vi "from string.vi"(8 "error in":errorcluster, 9 "data":string, 10 "version":string, 11 "TEC configuration in":refnum<class "TEC configuration.lvclass">) -> (0 "error out":errorcluster, 3 "TEC configuration out":refnum<class "TEC configuration.lvclass">)   [LabVIEW 2013, in "TEC configuration.lvclass"]
doc: "Provides an interface for loading a module configuration from a file or other serialized data source. It is recommended that all children of this class store data in two sets--data required for its own initialization, and any data required for parent initialization--and that each implementation uses the <b>Call Parent Method</b> primitive to de-serialize parent information. As a result, it is expected that every module configuration class calls <b>component configuration.lvclass:From String.vi</b>."
uses:
  TEC configuration.lvclass
  <vilib>/NI/Tag Bus Module Framework/channel/TBM channel.lvclass
  <vilib>/NI/Tag Bus Module Framework/module configuration/TBM module configuration.lvclass
  TEC configuration.lvclass/TEC configuration.ctl
  <vilib>/NI/Tag Bus Module Framework/root configuration/TBM configuration.lvclass
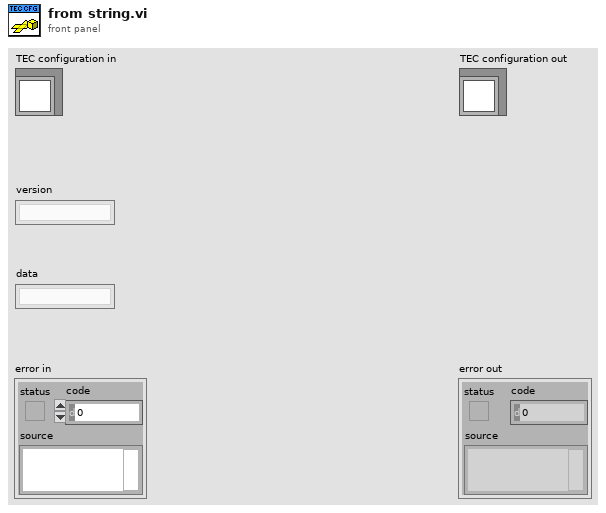
[diagram p1: front panel]
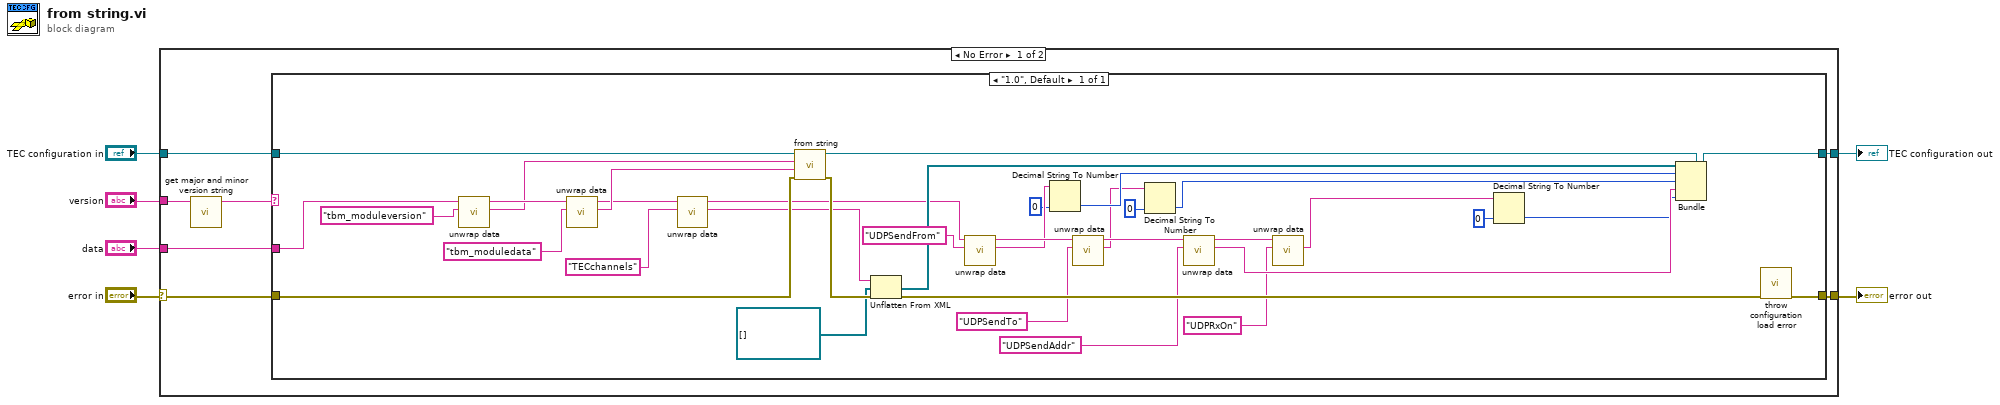
[diagram p0: block diagram]
diagram:
  n1 = case shown="No Error" "error in" {
    selector: "error in" -> [w7 w51]
    tunnel: "data" -> [w13 _]
    tunnel: "TEC configuration in" -> [w12 w50]
    tunnel: [w11 w50] -> w5
    tunnel: [w10 w51] -> w4
    tunnel: "version" -> [w9 _]
    frame No Error {
      n2 = call <vilib>:"get major and minor version string.vi"("full version"=w9) -> ("major.minor version"=w8:string)  [unwired: 10 in]
      n3 = case shown="\"1.0\", Default" w8 {
        tunnel: w13 -> [w44]
        tunnel: w7 -> [w43]
        tunnel: w12 -> [w49]
        tunnel: [w38] -> w11
        tunnel: [w46] -> w10
        frame "1.0", Default {
          n4 = call <vilib>:"unwrap data.vi"("identifier"="tbm_moduleversion" ("additional identifier"), "data to unwrap"=w44) -> ("unwrapped data"=w39:string, "remaining string"=w45:string)  [unwired: 8 in]
          n5 = call <vilib>:"unwrap data.vi"("identifier"="tbm_moduledata" ("additional identifier"), "data to unwrap"=w45) -> ("unwrapped data"=w41:string, "remaining string"=w34:string)  [unwired: 8 in]
          n6 = call <vilib>:"unwrap data.vi"("identifier"="TECchannels" ("additional identifier"), "data to unwrap"=w34) -> ("unwrapped data"=w32:string, "remaining string"=w28:string)  [unwired: 8 in]
          n7 = call-parent "from string.vi"("error in"=w43, "data"=w41, "version"=w39, "module configuration in"=w49) -> ("error out"=w47:errorcluster, "module configuration out"=w48:refnum<class "TEC configuration.lvclass">)  [unwired: 6 in]
          n8 = Unflatten From XML(xml string=w32, type=refnum<class "TBM channel.lvclass">[] [] ("channels"), error in (no error)=w47) -> (value=w35:refnum<class "TBM channel.lvclass">[], error out=w37:errorcluster)
          n9 = call <vilib>:"unwrap data.vi"("identifier"="UDPSendFrom" ("additional identifier"), "data to unwrap"=w28) -> ("unwrapped data"=w26:string, "remaining string"=w30:string)  [unwired: 8 in]
          n10 = Decimal String To Number(string=w26, default (0L)=u16 0 ("default (0 I32)")) -> (number=w19:u16)  [unwired: 1 in, 1 out]
          n11 = call <vilib>:"unwrap data.vi"("identifier"="UDPSendTo" ("additional identifier"), "data to unwrap"=w30) -> ("unwrapped data"=w18:string, "remaining string"=w31:string)  [unwired: 8 in]
          n12 = Decimal String To Number(string=w18, default (0L)=u16 0 ("default (0 I32)")) -> (number=w20:u16)  [unwired: 1 in, 1 out]
          n13 = call <vilib>:"unwrap data.vi"("identifier"="UDPSendAddr" ("additional identifier"), "data to unwrap"=w31) -> ("unwrapped data"=w22:string, "remaining string"=w29:string)  [unwired: 8 in]
          n14 = call <vilib>:"unwrap data.vi"("identifier"="UDPRxOn" ("additional identifier"), "data to unwrap"=w29) -> ("unwrapped data"=w17:string)  [unwired: 8 in, 1 out]
          n15 = Decimal String To Number(string=w17, default (0L)=u16 0 ("default (0 I32)")) -> (number=w21:u16)  [unwired: 1 in, 1 out]
          n16 = Bundle(cluster=w48, w35, w19, w20, w22, w21) -> (w38:refnum<class "TEC configuration.lvclass">)
          n17 = call <vilib>:"throw configuration load error.vi"("error in"=w37) -> ("error out"=w46:errorcluster)  [unwired: 10 in]
        }
      }
    }
    frame Error {
    }
  }
  "error out" <- w4
  "TEC configuration out" <- w5
